vi "Nearest.vi"(10 "Target":dbl[](array[numeric]), 11 "Pontos":dbl[][](array[numeric])) -> (2 "Nearest":dbl[](array[numeric]))   [LabVIEW 2017]
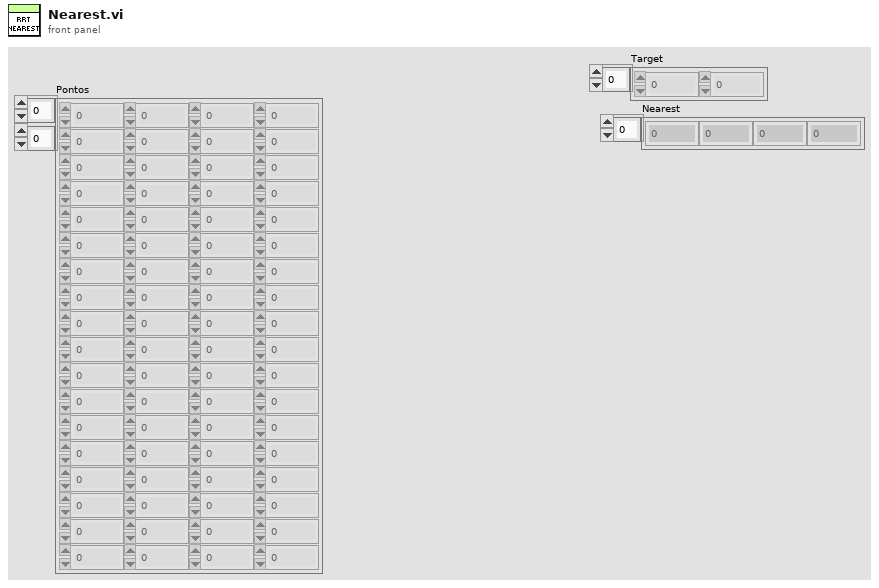
[diagram p1: front panel]
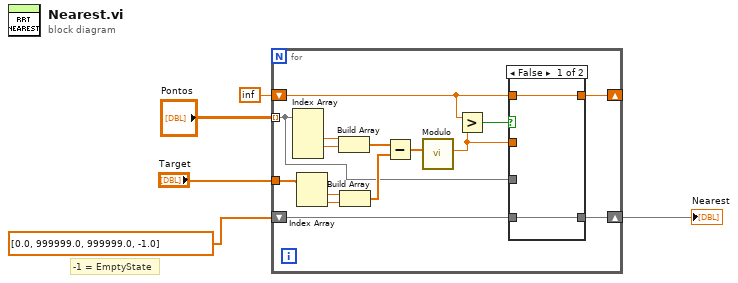
[diagram p0: block diagram]
diagram:
  # "-1 = EmptyState"
  n1 = for {
    tunnel: "Pontos" -> [w10] mode=indexing
    shift-right: [w14] -> _
    shift-left: inf -> [w13]
    tunnel: "Target" -> [w9]
    shift-right: [w7] -> w1
    shift-left: dbl[] [0.0, 999999.0, 999999.0, -1.0] ("Nearest 2") -> [w8]
    n2 = Index Array(array=w10) -> (element #2=w20:dbl, element #3=w19:dbl)  [unwired: 4 in, 2 out]
    n3 = Index Array(array=w9) -> (element #1=w12:dbl, element #2=w11:dbl)  [unwired: 2 in]
    n4 = Build Array(w20, w19) -> (w17:dbl[])
    n5 = Build Array(w12, w11) -> (w16:dbl[])
    n6 = Subtract(x=w17, y=w16) -> (x-y=w18:dbl[])
    n7 = call "Modulo.vi"("2D vector"=w18) -> ("Modulo"=w6:dbl)  [unwired: 10 in]
    n8 = Greater?(x=w13, y=w6) -> (0:w15:bool)
    n9 = case shown="False" w15 {
      tunnel: [w22 w23] -> w14
      tunnel: w13 -> [w22 _]
      tunnel: w10 -> [_ w24]
      tunnel: [w21 w24] -> w7
      tunnel: w8 -> [w21 _]
      tunnel: w6 -> [_ w23]
      frame False {
      }
      frame True {
      }
    }
  }
  "Nearest" <- w1
